vi "NEO VI Example.vi"() -> ()   [LabVIEW 2009]
panel:
  out "msg read?":bool
  out "sn":string
  out "DeviceType:":i32(ring)=65535 items=["NEODEVICE_BLUE"=1, "NEODEVICE_DW_VCAN"=4, "NEODEVICE_FIRE"=8, "NEODEVICE_VCAN3"=16, "NEODEVICE_YELLOW"=32, "NEODEVICE_ALL"=65535]
  out "Number Read:":i32
  out "Number Errors:":i32
  out "Error Info":string
  in  "Get Errors":bool
  out "Msgs":string
  in  "AutoRead":bool
  in  "Wait with Timeout":bool
  in  "Get Messages":bool
  in  "Data":u8[](array[numeric]) format="%.0x"
  in  "Transmit":bool
  in  "Number of \nData Bytes":i32(ring)=8 items=["0", "1", "2", "3", "4", "5", "6", "7", "8", "9", "10", "11"]
  in  "Send Extended ID":bool
  in  "Arb ID":u32 format="%.0x"
  in  "Network":T1(ring)
  in  "Tab Control":enum32{"Quick Set", "Advanced"}(tab)
  in  "Set Bit Rate":bool
  in  "Bit Rate":i32(ring)=20000 items=["20000"=20000, "33333"=33333, "50000"=50000, "62500"=62500, "83333"=83333, "100000"=100000, "125000"=125000, "250000"=250000, "500000"=500000, "800000"=800000, "1000000"=1000000]
  in  "CAN Channel":T2(ring)
  in  "Tab Control 2":enum32{"BLUE, VCAN2, Pro", "FIRE, Red, VCAN3"}(tab)
  in  "Send HS CAN information":bool
  in  "Set HS CAN 250":bool
  in  "Set HS CAN 500":bool
  in  "CNF3":u8 format="%.0x"
  in  "CNF2":u8 format="%.0x"
  in  "CNF1":u8 format="%.0x"
  out "Configuration":string
  in  "Get Configuration":bool
  in  "BRP":u16
  in  "Sync Jump Width":u8
  in  "Propagation Delay":u8
  in  "Phase Segment 2":u8
  in  "Phase Segment 1":u8
  in  "Set 3G Settings":bool
  in  "Get 3G settings":bool
  in  "Get DLL version":bool
  out "status":string
  in  "Close Open Device":bool
  in  "Open First Device":bool
  # "Connection"
  # "Baud Rate"
  # "Transmit Message"
  # "Data in Hex"
  # "Receive Message"
  # "Tip: Use neoVI explorer to get the proper CNFs.\nValueCAN CNFs are different than neoVI due to\ndifferent CAN Chip speeds."
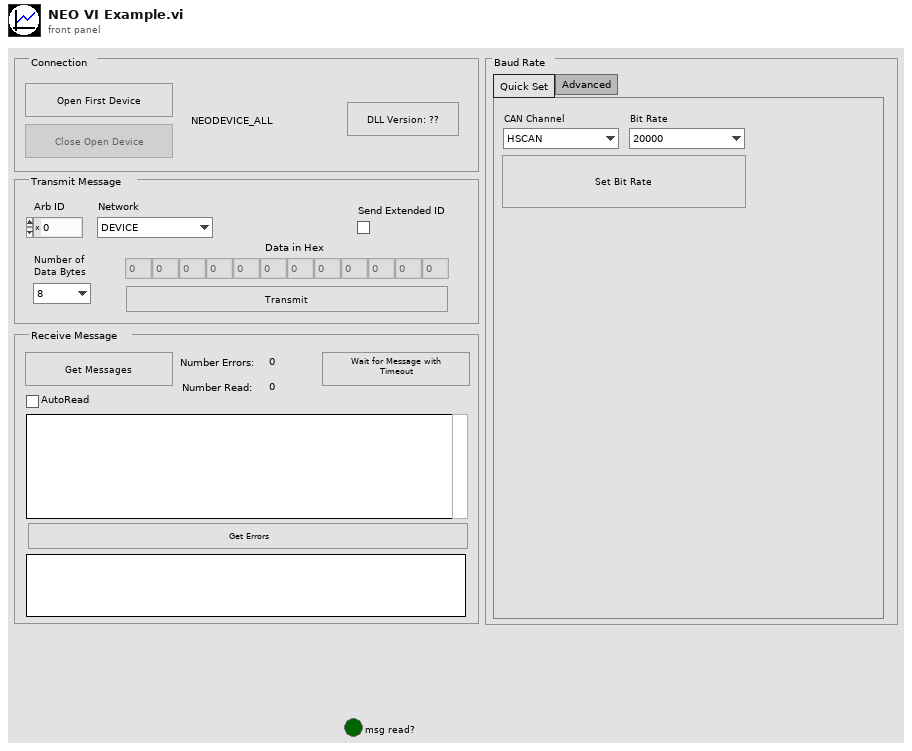
[diagram p1: front panel]
types:
  T1 = enum16{"DEVICE", "HSCAN", "MSCAN", "SWCAN", "LSFTCAN", "FORDSCP", "J1708", "JVPW", "ISO", "FIRE_HSCAN2", "FIRE_MSCAN1", "FIRE_HSCAN3", "FIRE_LIN2", "FIRE_LIN3", "FIRE_LIN4"}
  T2 = enum16{"HSCAN", "MSCAN", "SWCAN", "LSFTCAN", "HSCAN2", "HSCAN3"}
  T3 = enum8{"Enabled", "Disabled", "Disabled and Grayed Out"}
  T4 = cluster{"DeviceType":i32, "Handle":i32, "NumberOfClients":i32, "SerialNumber":i32, "MaxAllowedClients":i32}[]
  T5 = cluster{"DeviceType":i32, "Handle":i32, "NumberOfClients":i32, "SerialNumber":i32, "MaxAllowedClients":i32}
  T6 = typedef "ctl FireSetting.ctl" = cluster{"can 1":cluster{"Mode":u8, "SetBaudrate":u8, "Baudrate":u8, "NetworkType":u8, "TqSeg1":u8, "TqSeg2":u8, "TqProp":u8, "TqSync":u8, "BRP":u16, "auto_baud":u16}, "can 2":cluster{"Mode":u8, "SetBaudrate":u8, "Baudrate":u8, "NetworkType":u8, "TqSeg1":u8, "TqSeg2":u8, "TqProp":u8, "TqSync":u8, "BRP":u16, "auto_baud":u16}, "can 3":cluster{"Mode":u8, "SetBaudrate":u8, "Baudrate":u8, "NetworkType":u8, "TqSeg1":u8, "TqSeg2":u8, "TqProp":u8, "TqSync":u8, "BRP":u16, "auto_baud":u16}, "can 4":cluster{"Mode":u8, "SetBaudrate":u8, "Baudrate":u8, "NetworkType":u8, "TqSeg1":u8, "TqSeg2":u8, "TqProp":u8, "TqSync":u8, "BRP":u16, "auto_baud":u16}, "swcan":cluster{"Mode":u8, "SetBaudrate":u8, "Baudrate":u8, "NetworkType":u8, "TqSeg1":u8, "TqSeg2":u8, "TqProp":u8, "TqSync":u8, "BRP":u16, "high_speed_auto_switch":u16, "auto_baud":u16}, "lsftcan":cluster{"Mode":u8, "SetBaudrate":u8, "Baudrate":u8, "NetworkType":u8, "TqSeg1":u8, "TqSeg2":u8, "TqProp":u8, "TqSync":u8, "BRP":u16, "auto_baud":u16}, "lin 1":cluster{"Baudrate":u32, "spbrg":u16, "brgh":u16, "MasterResistor":u8, "Mode":u8}, "lin 2":cluster{"Baudrate":u32, "spbrg":u16, "brgh":u16, "MasterResistor":u8, "Mode":u8}, "lin 3":cluster{"Baudrate":u32, "spbrg":u16, "brgh":u16, "MasterResistor":u8, "Mode":u8}, "lin 4":cluster{"Baudrate":u32, "spbrg":u16, "brgh":u16, "MasterResistor":u8, "Mode":u8}, "cgi_enable":u16, "cgi_baud":u16, "cgi_tx_ifs_bit_times":u16, "cgi_rx_ifs_bit_times":u16, "cgi_chksum_enable":u16, "network_enalbes":u16, "network_enabled_on_boot":u16, "pwm_man_timeout":u16, "pwm_man_enable":u16, "misc_io_initial_ddr":u16, "misc_io_initial_latch":u16, "misc_io_analog_enable":u16, "misc_io_report_period":u16, "misc_io_on_report_events":u16, "ain_sample_period":u16, "ain_threshold":u16, "iso15765_separation_time_offset":u16, "iso9141_kwp_enable":u16, "ISO9141_Settings":cluster{"Baudrate":u32, "spbrg":u16, "brgh":u16, "ISO9141_KEYWORD2000_INIT_STEP":cluster{"time_500us":u16, "k":u16, "l":u16}, "init_step_count":u8, "p2_500us":u16, "p3_500us":u16, "p4_500us":u16, "chksum_enabled":u16}, "perf_en":u16, "iso_parity":u16, "iso_msg_termination":u16, "iso_tester_pullup_enable":u16, "network_enables_2":u16, "ISO9141__Settings2":cluster{"Baudrate":u32, "spbrg":u16, "brgh":u16, "ISO9141_KEYWORD2000_INIT_STEP":cluster{"time_500us":u16, "k":u16, "l":u16}, "init_step_count":u8, "p2_500us":u16, "p3_500us":u16, "p4_500us":u16, "chksum_enabled":u16}, "iso_parity_2":u16, "iso_msg_termination_2":u16, "ISO9141_Settings_3":cluster{"Baudrate":u32, "spbrg":u16, "brgh":u16, "ISO9141_KEYWORD2000_INIT_STEP":cluster{"time_500us":u16, "k":u16, "l":u16}, "init_step_count":u8, "p2_500us":u16, "p3_500us":u16, "p4_500us":u16, "chksum_enabled":u16}, "iso_parity_3":u16, "iso_msg_termination_3":u16, "ISO9141_Settings_4":cluster{"Baudrate":u32, "spbrg":u16, "brgh":u16, "ISO9141_KEYWORD2000_INIT_STEP":cluster{"time_500us":u16, "k":u16, "l":u16}, "init_step_count":u8, "p2_500us":u16, "p3_500us":u16, "p4_500us":u16, "chksum_enabled":u16}, "iso_parity_4":u16, "iso_msg_termination_4":u16}
  T7 = typedef "ctl SVCANSetting.ctl" = cluster{"can 1":cluster{"Mode":u8, "SetBaudrate":u8, "Baudrate":u8, "NetworkType":u8, "TqSeg1":u8, "TqSeg2":u8, "TqProp":u8, "TqSync":u8, "BRP":u16, "auto_baud":u16}, "can 2":cluster{"Mode":u8, "SetBaudrate":u8, "Baudrate":u8, "NetworkType":u8, "TqSeg1":u8, "TqSeg2":u8, "TqProp":u8, "TqSync":u8, "BRP":u16, "auto_baud":u16}, "network_enables":u16, "network_enabled_on_boot":u16, "iso15765_separation_time_offset":i16, "perf_en":u16, "misc_io_initial_ddr":u16, "misc_io_initial_latach":u16, "misc_io_report_period":u16, "misc_io_on_report_events":u16}
  T8 = typedef "ctl spymessage.ctl" = cluster{"StatusBitField":u32, "StatusBitField2":u32, "TimeHardware":u32, "TimeHardware2":u32, "TimeSystem":u32, "TimeSystem2":u32, "TimeStampHardwareID":u8, "TimeStampHardwareID2":u8, "NetworkID":u8, "NodeID":u8, "Protocol":u8, "MessagePieceID":u8, "ColorID":u8, "NumberBytesHeader":u8, "NumberBytesData":u8, "DescriptionID":u16, "ArbIDOrHeader":u32, "Data [8]":u8[], "AckBytes [8]":u8[], "Value":sgl, "MiscData":u8}
  T9 = enum16{"No Error", "Critical", "Important", "Warning", "Unknown"}
  T10 = cluster{"ErrorNumber":i32, "short":string, "long":string}
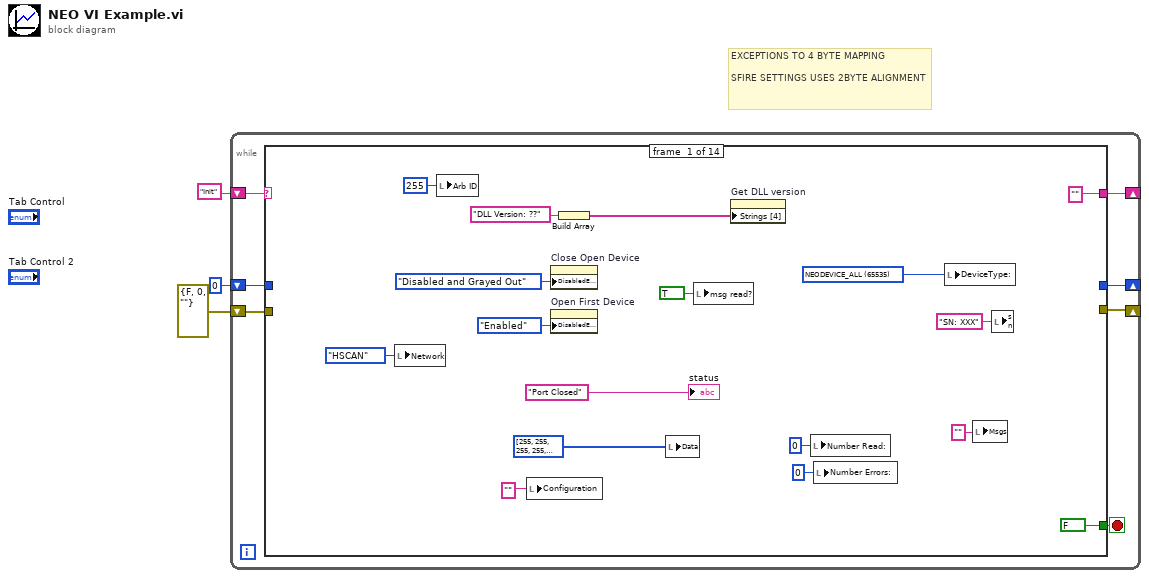
[diagram p0: block diagram]
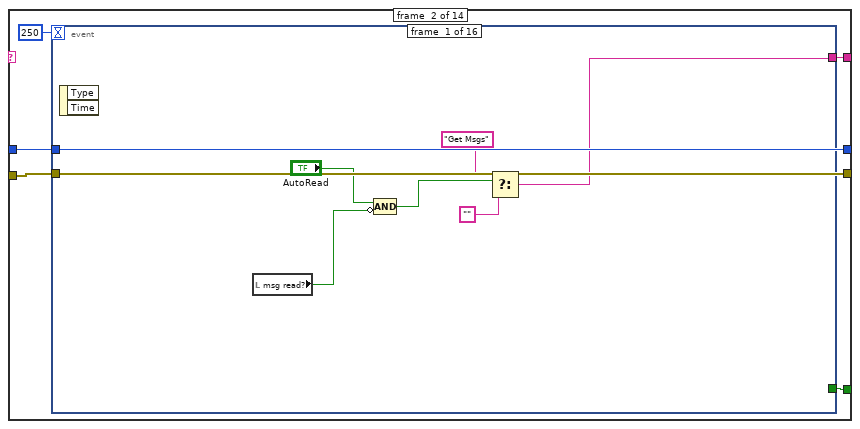
[diagram p2: hidden frame]
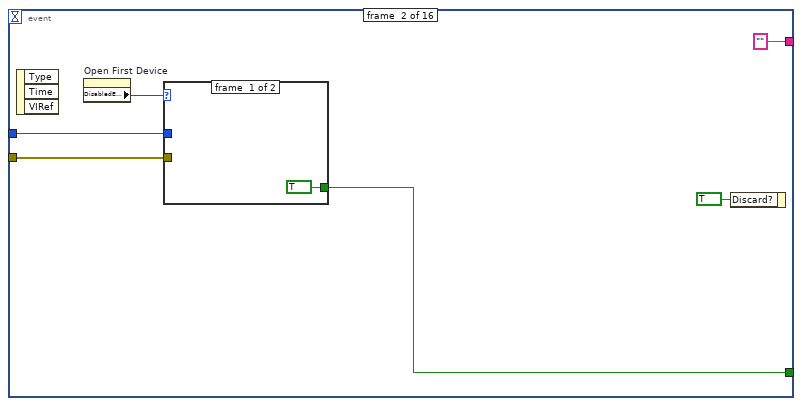
[diagram p3: hidden frame]
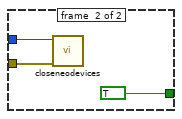
[diagram p4: hidden frame]
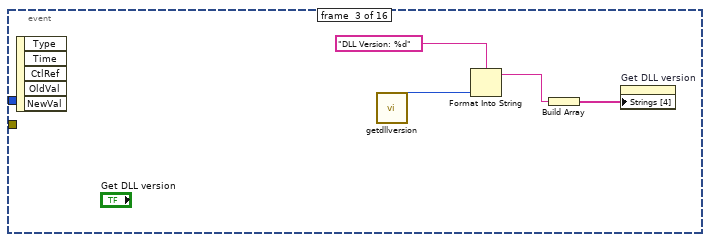
[diagram p5: hidden frame]
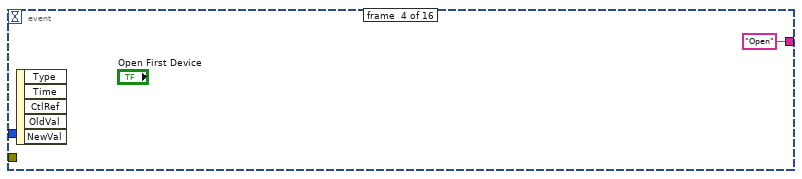
[diagram p6: hidden frame]
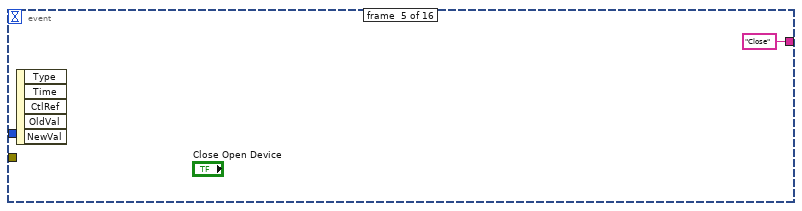
[diagram p7: hidden frame]
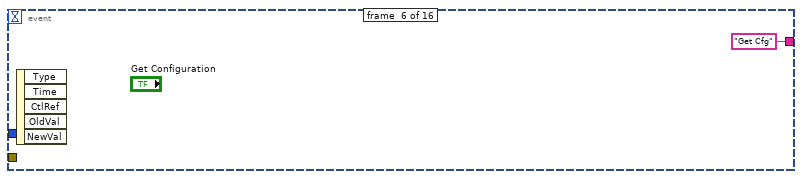
[diagram p8: hidden frame]
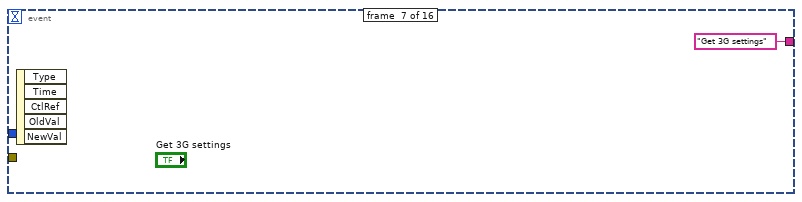
[diagram p9: hidden frame]
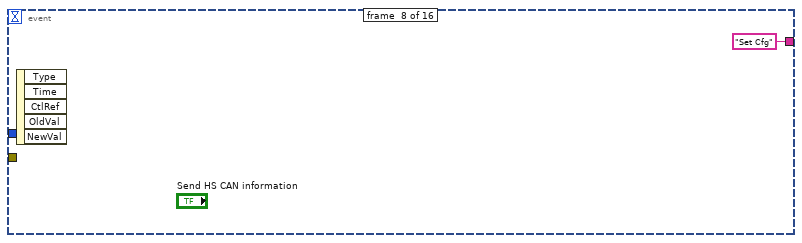
[diagram p10: hidden frame]
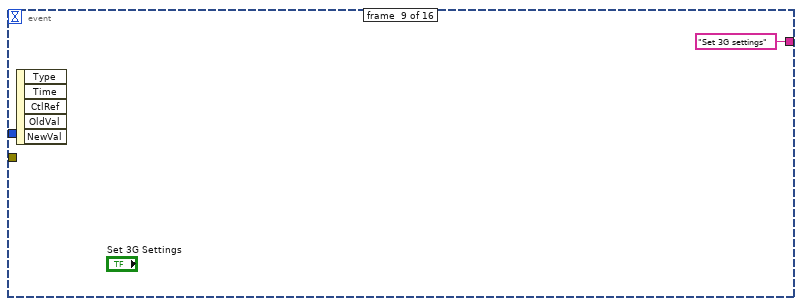
[diagram p11: hidden frame]
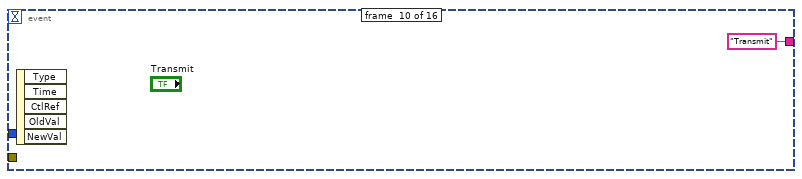
[diagram p12: hidden frame]
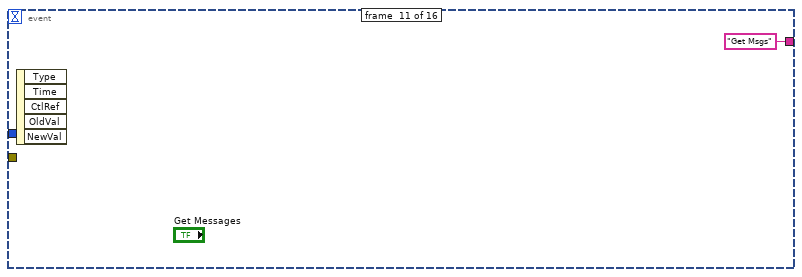
[diagram p13: hidden frame]
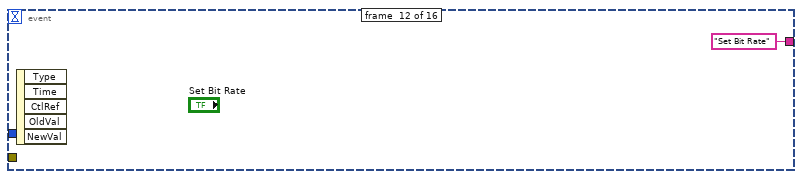
[diagram p14: hidden frame]
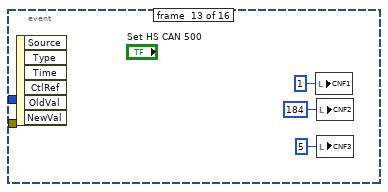
[diagram p15: hidden frame]
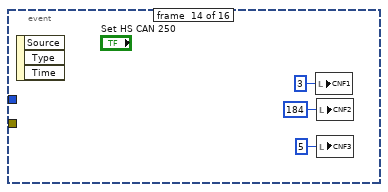
[diagram p16: hidden frame]
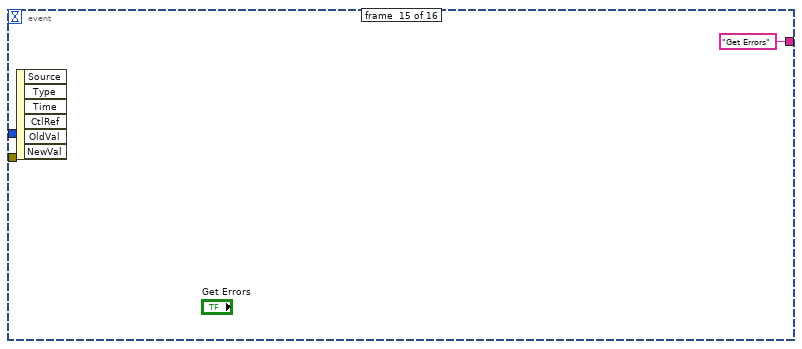
[diagram p17: hidden frame]
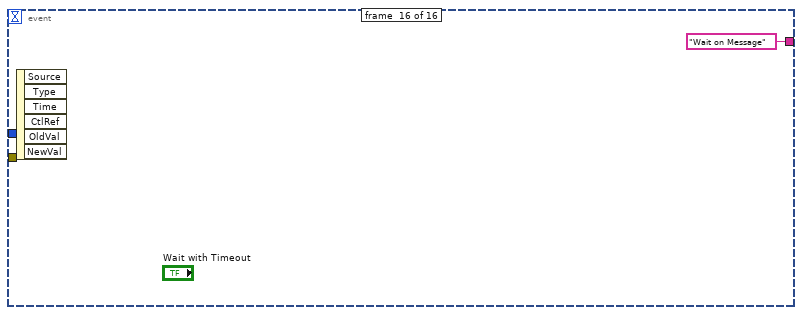
[diagram p18: hidden frame]
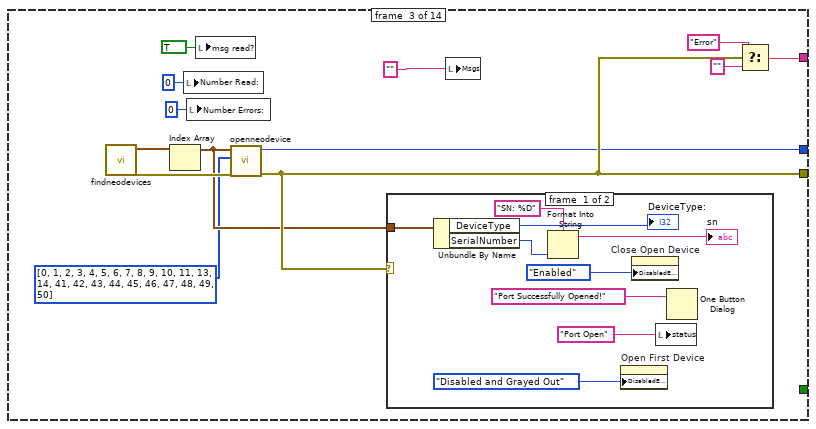
[diagram p19: hidden frame]
diagram:
  # "EXCEPTIONS TO 4 BYTE MAPPING\n\nSFIRE SETTINGS USES 2BYTE ALIGNMENT"
  n1 = while {
    shift-right: [w8] -> _
    shift-left: "Init" -> [w9]
    shift-right: [w7] -> _
    shift-left: 0 ("hObject") -> [w6]
    shift-right: [w5] -> _
    shift-left: errorcluster {"status"=FALSE, "code"=0, "source"=""} ("error out") -> [w4]
    stop <- w10 stop-if-true
    n2 = case shown="\"Open\"" w9 {
      tunnel: [FALSE w32 _ _ _ _ _ _ _ _ _ _ _ _] -> w10
      tunnel: ["" w31 w82 w98 "" ("f") w132 w151 w173 w213 w253 w275 "" ("f") _ _] -> w8
      tunnel: [_ w29 w75 _ w111 w129 w159 w174 w211 w248 w272 0 ("hObject") w291 w318] -> w7
      tunnel: w6 -> [_ w29 _ w94 w110 w142 w158 w179 w204 w258 w279 _ w292 w325]
      tunnel: [_ w28 w79 w95 w112 w128 w152 w175 w212 w254 w270 errorcluster {"status"=FALSE, "code"=0, "source"=""} ("error out") w288 w319] -> w5
      tunnel: w4 -> [_ w28 _ w93 w113 w143 w160 w178 w205 w259 w280 _ w293 w324]
      frame #0 {
        w19 = 65535 items=["NEODEVICE_BLUE"=1, "NEODEVICE_DW_VCAN"=4, "NEODEVICE_FIRE"=8, "NEODEVICE_VCAN3"=16, "NEODEVICE_YELLOW"=32, "NEODEVICE_ALL"=65535] ("DeviceType:")
        n3 = local write "Network"(T1."HSCAN" ("Network")) -> ()
        n4 = local write "Arb ID"(u32 255 ("Arb ID")) -> ()
        n5 = local write "Configuration"("") -> ()
        n6 = property on="Close Open Device" class="Bool"("DisabledEnum"=T3."Disabled and Grayed Out" ("Disabled")) -> ()  [unwired: 2 in, 2 out]
        n7 = property on="Open First Device" class="Bool"("DisabledEnum"=T3."Enabled" ("Disabled")) -> ()  [unwired: 2 in, 2 out]
        n8 = Build Array("DLL Version: ??") -> (w25:string[])
        n9 = local write "Data"(u16[] [255, 255, 255, 255, 255, 255, 255, 255, 255, 255, 255, 255] ("Array")) -> ()
        n10 = local write "msg read?"(TRUE ("msg read?")) -> ()
        n11 = property on="Get DLL version" class="Bool"("Strings [4]"=w25) -> ()  [unwired: 2 in, 2 out]
        n12 = local write "Number Read:"(0 ("Number Read:")) -> ()
        n13 = local write "Number Errors:"(0 ("Number Errors:")) -> ()
        n14 = local write "DeviceType:"(w19) -> ()
        n15 = local write "Msgs"("" ("Msgs")) -> ()
        n16 = local write "sn"("SN: XXX" ("sn")) -> ()
        "status" <- "Port Closed" ("status")
      }
      frame #1 {
        n17 = event shown="[3] \"Open First Device\": Value Change" {
          selector: _ -> [_ _ _ _ _ _ _ _ _ _ _ _ _ _ _ _]
          dyn-events: _ -> [_ _ _ _ _ _ _ _ _ _ _ _ _ _ _ _]
          timeout: 250 -> [_ _ _ _ _ _ _ _ _ _ _ _ _ _ _ _]
          tunnel: [_ w39 _ _ _ _ _ _ _ _ _ _ _ _ _ _] -> w32
          tunnel: [w36 "" _ "Open" "Close" "Get Cfg" "Get 3G settings" "Set Cfg" "Set 3G settings" "Transmit" "Get Msgs" "Set Bit Rate" _ _ "Get Errors" ("f") "Wait on Message" ("f")] -> w31
          tunnel: w29 -> [_ w42 _ _ _ _ _ _ _ _ _ _ _ _ _ _]
          tunnel: w28 -> [_ w41 _ _ _ _ _ _ _ _ _ _ _ _ _ _]
          event #0 {
            n18 = event-data() -> ()  [unwired: 3 out]
            n19 = local read "msg read?"() -> (w33:bool)
            n20 = Compound Arithmetic op=AND("AutoRead", invert w33) -> (w34:bool)
            n21 = Select(t="Get Msgs", s=w34, f="") -> (s? t:f=w36:string)
          }
          event #1 {
            n22 = event-data() -> ()  [unwired: 4 out]
            n23 = property on="Open First Device" class="Bool"() -> ("DisabledEnum"=w40:T3)  [unwired: 2 in, 2 out]
            n24 = case shown="\"Enabled\", Default" w40 {
              tunnel: w42 -> [_ w48]
              tunnel: w41 -> [_ w47]
              tunnel: [TRUE TRUE] -> w39
              frame #0 {
              }
              frame #1 {
                n25 = call "closeneodevices.vi"("error in (no error)"=w47, "hObject"=w48) -> ()  [unwired: 1 in, 9 out]
              }
            }
            n26 = event-data("Discard?"=TRUE) -> ()  [unwired: 1 in, 1 out]
          }
          event #2 {
            n27 = event-data() -> ()  [unwired: 6 out]
            n28 = call "getdllversion.vi"() -> ("DLLVersion"=w52:i32)  [unwired: 1 in, 10 out]
            n29 = Format Into String(format string="DLL Version: %d", w52) -> (resulting string=w50:string)  [unwired: 2 in, 1 out]
            n30 = Build Array(w50) -> (w49:string[])
            n31 = property on="Get DLL version" class="Bool"("Strings [4]"=w49) -> ()  [unwired: 2 in, 2 out]
          }
          event #3 {
            n32 = event-data() -> ()  [unwired: 6 out]
          }
          event #4 {
            n33 = event-data() -> ()  [unwired: 6 out]
          }
          event #5 {
            n34 = event-data() -> ()  [unwired: 6 out]
          }
          event #6 {
            n35 = event-data() -> ()  [unwired: 6 out]
          }
          event #7 {
            n36 = event-data() -> ()  [unwired: 6 out]
          }
          event #8 {
            n37 = event-data() -> ()  [unwired: 6 out]
          }
          event #9 {
            n38 = event-data() -> ()  [unwired: 6 out]
          }
          event #10 {
            n39 = event-data() -> ()  [unwired: 6 out]
          }
          event #11 {
            n40 = event-data() -> ()  [unwired: 6 out]
          }
          event #12 {
            n41 = event-data() -> ()  [unwired: 7 out]
            n42 = local write "CNF1"(u8 1 ("CNF1")) -> ()
            n43 = local write "CNF2"(u8 184 ("CNF2")) -> ()
            n44 = local write "CNF3"(u8 5 ("CNF3")) -> ()
          }
          event #13 {
            n45 = event-data() -> ()  [unwired: 4 out]
            n46 = local write "CNF1"(u8 3 ("CNF1")) -> ()
            n47 = local write "CNF2"(u8 184 ("CNF2")) -> ()
            n48 = local write "CNF3"(u8 5 ("CNF3")) -> ()
          }
          event #14 {
            n49 = event-data() -> ()  [unwired: 7 out]
          }
          event #15 {
            n50 = event-data() -> ()  [unwired: 7 out]
          }
        }
      }
      frame #2 {
        w70 = i8[] [0, 1, 2, 3, 4, 5, 6, 7, 8, 9, 10, 11, 13, 14, 41, 42, 43, 44, 45, 46, 47, 48, 49, 50] items=["NETID_DEVICE"=0, "NETID_HSCAN"=1, "NETID_MSCAN"=2, "NETID_SWCAN"=3, "NETID_LSFTCAN"=4, "NETID_FORDSCP"=5, "NETID_J1708"=6, "NETID_AUX"=7, "NETID_JVPW"=8, "NETID_ISO_LIN"=9, "NETID_ISOPIC"=10, "NETID_MAIN51"=11, "NETID_SCI"=13, "NETID_ISO2"=14, "NETID_FIRE_HSCAN1"=41, "NETID_FIRE_HSCAN2"=42, "NETID_FIRE_MSCAN1"=43, "NETID_FIRE_MSCAN2_HSCAN3"=44, "NETID_FIRE_SWCAN"=45, "NETID_FIRE_LSFT"=46, "NETID_FIRE_LIN1"=47, "NETID_FIRE_LIN2"=48, "NETID_FIRE_LIN3"=49, "NETID_FIRE_LIN4"=50] ("bNetworkIDs")
        n51 = call "findneodevices.vi"() -> ("error out"=w77:errorcluster, "NeoDevices {}"=w78:T4)  [unwired: 3 in, 7 out]
        n52 = Index Array(array=w78) -> (element=w76:T5)  [unwired: 1 in]
        n53 = local write "Number Read:"(0 ("Number Read:")) -> ()
        n54 = local write "Number Errors:"(0 ("Number Errors:")) -> ()
        n55 = local write "msg read?"(TRUE ("msg read?")) -> ()
        n56 = call "openneodevice.vi"("error in (no error)"=w77, "bNetworkIDs"=w70, "NeoDevice{}"=w76) -> ("error out"=w79:errorcluster, "hObject"=w75:i32)  [unwired: 2 in, 5 out]
        n57 = case shown="No Error" w79 {
          tunnel: w76 -> [w87 _]
          frame #0 {
            n58 = Unbundle By Name(w87) -> ("DeviceType"=→"DeviceType:":i32, "SerialNumber"=w85:i32)
            n59 = Format Into String(format string="SN: %D", w85) -> (resulting string=→"sn":string)  [unwired: 2 in, 1 out]
            n60 = property on="Open First Device" class="Bool"("DisabledEnum"=T3."Disabled and Grayed Out" ("Disabled")) -> ()  [unwired: 2 in, 2 out]
            n61 = property on="Close Open Device" class="Bool"("DisabledEnum"=T3."Enabled" ("Disabled")) -> ()  [unwired: 2 in, 2 out]
            n62 = local write "status"("Port Open" ("status")) -> ()
            n63 = One Button Dialog(message="Port Successfully Opened!") -> ()  [unwired: 2 out]
          }
          frame #1 {
          }
        }
        n64 = local write "Msgs"("" ("Msgs")) -> ()
        n65 = Select(t="Error", s=w79, f="") -> (s? t:f=w82:string)
      }
      frame #3 {
        n66 = local write "msg read?"(TRUE ("msg read?")) -> ()
        n67 = call "closeneodevices.vi"("error in (no error)"=w93, "hObject"=w94) -> ("error out"=w95:errorcluster)  [unwired: 1 in, 8 out]
        n68 = case shown="No Error" w95 {
          frame #0 {
            w100 = 65535 items=["NEODEVICE_BLUE"=1, "NEODEVICE_DW_VCAN"=4, "NEODEVICE_FIRE"=8, "NEODEVICE_VCAN3"=16, "NEODEVICE_YELLOW"=32, "NEODEVICE_ALL"=65535] ("DeviceType:")
            n69 = local write "sn"("SN: XXX" ("sn")) -> ()
            n70 = property on="Open First Device" class="Bool"("DisabledEnum"=T3."Enabled" ("Disabled")) -> ()  [unwired: 2 in, 2 out]
            n71 = local write "status"("Port Closed" ("status")) -> ()
            n72 = local write "DeviceType:"(w100) -> ()
            n73 = property on="Close Open Device" class="Bool"("DisabledEnum"=T3."Disabled and Grayed Out" ("Disabled")) -> ()  [unwired: 2 in, 2 out]
          }
          frame #1 {
          }
        }
        n74 = Select(t="Error", s=w95, f="") -> (s? t:f=w98:string)
      }
      frame #4 {
        n75 = call "getconfiguration.vi"("error in (no error)"=w113, "hObject"=w110) -> ("error out"=w112:errorcluster, "pINumBytes"=w105:i32, "pData"=w109:u8[], "hObject Out"=w111:i32)  [unwired: 6 out]
        n76 = for {
          N: w105 -> [_]
          tunnel: w109 -> [w118] mode=indexing
          tunnel: "Byte %d: %d " ("format string") -> [w120]
          shift-right: [w114] -> w106
          shift-left: "" -> [w117]
          i -> [w119]
          n77 = Format Into String(format string=w120, w119, w118) -> (resulting string=w116:string)  [unwired: 2 in, 1 out]
          n78 = Concatenate Strings(w117, w116, "\r") -> (w114:string)
        }
        "Configuration" <- w106
      }
      frame #5 {
        n79 = call "getconfiguration.vi"("error in (no error)"=w143, "hObject"=w142) -> ("error out"=w141:errorcluster, "pData"=w136:u8[], "hObject Out"=w140:i32)  [unwired: 7 out]
        n80 = Replace Array Subset(array=w136, new element #1="CNF1", index #1=522 ("index"), new element #2="CNF2", index #2=521 ("index"), new element #3="CNF3", index #3=520 ("index")) -> (w135:u8[])
        n81 = call "sendconfiguration.vi"("error in (no error)"=w141, "pData"=w135, "hObject"=w140) -> ("error out"=w131:errorcluster, "hObject Out"=w130:i32)  [unwired: 7 out]
        n82 = call "getconfiguration.vi"("error in (no error)"=w131, "hObject"=w130) -> ("error out"=w128:errorcluster, "pData"=w125:u8[], "hObject Out"=w129:i32)  [unwired: 7 out]
        n83 = for {
          tunnel: w125 -> [w148] mode=indexing
          tunnel: "Byte %d: %d " ("format string") -> [w150]
          shift-right: [w144] -> w124
          shift-left: "" -> [w147]
          i -> [w149]
          n84 = Format Into String(format string=w150, w149, w148) -> (resulting string=w146:string)  [unwired: 2 in, 1 out]
          n85 = Concatenate Strings(w147, w146, "\r") -> (w144:string)
        }
        n86 = local write "Configuration"(w124) -> ()
        n87 = Select(t="Error", s=w128, f="") -> (s? t:f=w132:string)
      }
      frame #6 {
        n88 = case shown="\"HSCAN3\"" "CAN Channel" {
          tunnel: [_ w161 w162 w163 w164 w165 w166] -> w155
          frame #0 {
          }
          frame #1 {
            w161 = i8 1 items=["NETID_DEVICE"=0, "NETID_HSCAN"=1, "NETID_MSCAN"=2, "NETID_SWCAN"=3, "NETID_LSFTCAN"=4, "NETID_FORDSCP"=5, "NETID_J1708"=6, "NETID_AUX"=7, "NETID_JVPW"=8, "NETID_ISO_LIN"=9, "NETID_ISOPIC"=10, "NETID_MAIN51"=11, "NETID_SCI"=13, "NETID_ISO2"=14, "NETID_FIRE_HSCAN1"=41, "NETID_FIRE_HSCAN2"=42, "NETID_FIRE_MSCAN1"=43, "NETID_FIRE_MSCAN2_HSCAN3"=44, "NETID_FIRE_SWCAN"=45, "NETID_FIRE_LSFT"=46, "NETID_FIRE_LIN1"=47, "NETID_FIRE_LIN2"=48, "NETID_FIRE_LIN3"=49, "NETID_FIRE_LIN4"=50] ("NetworkID")
          }
          frame #2 {
            w162 = i8 2 items=["NETID_DEVICE"=0, "NETID_HSCAN"=1, "NETID_MSCAN"=2, "NETID_SWCAN"=3, "NETID_LSFTCAN"=4, "NETID_FORDSCP"=5, "NETID_J1708"=6, "NETID_AUX"=7, "NETID_JVPW"=8, "NETID_ISO_LIN"=9, "NETID_ISOPIC"=10, "NETID_MAIN51"=11, "NETID_SCI"=13, "NETID_ISO2"=14, "NETID_FIRE_HSCAN1"=41, "NETID_FIRE_HSCAN2"=42, "NETID_FIRE_MSCAN1"=43, "NETID_FIRE_MSCAN2_HSCAN3"=44, "NETID_FIRE_SWCAN"=45, "NETID_FIRE_LSFT"=46, "NETID_FIRE_LIN1"=47, "NETID_FIRE_LIN2"=48, "NETID_FIRE_LIN3"=49, "NETID_FIRE_LIN4"=50] ("NetworkID")
          }
          frame #3 {
            w163 = i8 3 items=["NETID_DEVICE"=0, "NETID_HSCAN"=1, "NETID_MSCAN"=2, "NETID_SWCAN"=3, "NETID_LSFTCAN"=4, "NETID_FORDSCP"=5, "NETID_J1708"=6, "NETID_AUX"=7, "NETID_JVPW"=8, "NETID_ISO_LIN"=9, "NETID_ISOPIC"=10, "NETID_MAIN51"=11, "NETID_SCI"=13, "NETID_ISO2"=14, "NETID_FIRE_HSCAN1"=41, "NETID_FIRE_HSCAN2"=42, "NETID_FIRE_MSCAN1"=43, "NETID_FIRE_MSCAN2_HSCAN3"=44, "NETID_FIRE_SWCAN"=45, "NETID_FIRE_LSFT"=46, "NETID_FIRE_LIN1"=47, "NETID_FIRE_LIN2"=48, "NETID_FIRE_LIN3"=49, "NETID_FIRE_LIN4"=50] ("NetworkID")
          }
          frame #4 {
            w164 = i8 4 items=["NETID_DEVICE"=0, "NETID_HSCAN"=1, "NETID_MSCAN"=2, "NETID_SWCAN"=3, "NETID_LSFTCAN"=4, "NETID_FORDSCP"=5, "NETID_J1708"=6, "NETID_AUX"=7, "NETID_JVPW"=8, "NETID_ISO_LIN"=9, "NETID_ISOPIC"=10, "NETID_MAIN51"=11, "NETID_SCI"=13, "NETID_ISO2"=14, "NETID_FIRE_HSCAN1"=41, "NETID_FIRE_HSCAN2"=42, "NETID_FIRE_MSCAN1"=43, "NETID_FIRE_MSCAN2_HSCAN3"=44, "NETID_FIRE_SWCAN"=45, "NETID_FIRE_LSFT"=46, "NETID_FIRE_LIN1"=47, "NETID_FIRE_LIN2"=48, "NETID_FIRE_LIN3"=49, "NETID_FIRE_LIN4"=50] ("NetworkID")
          }
          frame #5 {
            w165 = i8 42 items=["NETID_DEVICE"=0, "NETID_HSCAN"=1, "NETID_MSCAN"=2, "NETID_SWCAN"=3, "NETID_LSFTCAN"=4, "NETID_FORDSCP"=5, "NETID_J1708"=6, "NETID_AUX"=7, "NETID_JVPW"=8, "NETID_ISO_LIN"=9, "NETID_ISOPIC"=10, "NETID_MAIN51"=11, "NETID_SCI"=13, "NETID_ISO2"=14, "NETID_FIRE_HSCAN1"=41, "NETID_FIRE_HSCAN2"=42, "NETID_FIRE_MSCAN1"=43, "NETID_FIRE_MSCAN2_HSCAN3"=44, "NETID_FIRE_SWCAN"=45, "NETID_FIRE_LSFT"=46, "NETID_FIRE_LIN1"=47, "NETID_FIRE_LIN2"=48, "NETID_FIRE_LIN3"=49, "NETID_FIRE_LIN4"=50] ("NetworkID")
          }
          frame #6 {
            w166 = i8 44 items=["NETID_DEVICE"=0, "NETID_HSCAN"=1, "NETID_MSCAN"=2, "NETID_SWCAN"=3, "NETID_LSFTCAN"=4, "NETID_FORDSCP"=5, "NETID_J1708"=6, "NETID_AUX"=7, "NETID_JVPW"=8, "NETID_ISO_LIN"=9, "NETID_ISOPIC"=10, "NETID_MAIN51"=11, "NETID_SCI"=13, "NETID_ISO2"=14, "NETID_FIRE_HSCAN1"=41, "NETID_FIRE_HSCAN2"=42, "NETID_FIRE_MSCAN1"=43, "NETID_FIRE_MSCAN2_HSCAN3"=44, "NETID_FIRE_SWCAN"=45, "NETID_FIRE_LSFT"=46, "NETID_FIRE_LIN1"=47, "NETID_FIRE_LIN2"=48, "NETID_FIRE_LIN3"=49, "NETID_FIRE_LIN4"=50] ("NetworkID")
          }
        }
        n89 = call "setbitrate.vi"("error in (no error)"=w160, "NetworkID"=w155, "BitRate"="Bit Rate", "hObject"=w158) -> ("error out"=w152:errorcluster, "hObject Out"=w159:i32)  [unwired: 6 out]
        n90 = Select(t="Error", s=w152, f="") -> (s? t:f=w151:string)
      }
      frame #7 {
        n91 = local read "DeviceType:"() -> (w167:i32)
        n92 = case shown="16" w167 {
          tunnel: w179 -> [w181 w192 w202]
          tunnel: w178 -> [w182 w191 w201]
          tunnel: [w182 w190 w200] -> w175
          tunnel: [w181 w189 w199] -> w174
          tunnel: [_ w187 w197] -> w172
          tunnel: [_ w186 w196] -> w171
          tunnel: [_ w185 w195] -> w170
          tunnel: [_ w184 w194] -> w169
          tunnel: [_ w183 w193] -> w168
          frame #0 {
            n93 = One Button Dialog(message="Problem reading configuration, unsupported device") -> ()  [unwired: 2 out]
          }
          frame #1 {
            n94 = call "getfiresettings.vi"("error in (no error)"=w191, "hObject"=w192) -> ("error out"=w190:errorcluster, "pSettings"=w188:T6, "hObject Out"=w189:i32)  [unwired: 7 out]
            n95 = Unbundle By Name(w188) -> ("can 1.TqSeg1"=w187:u8, "can 1.TqSeg2"=w186:u8, "can 1.TqProp"=w185:u8, "can 1.TqSync"=w184:u8, "can 1.BRP"=w183:u16)
          }
          frame #2 {
            n96 = call "getvcan3setting.vi"("error in (no error)"=w201, "hObject"=w202) -> ("error out"=w200:errorcluster, "SVCAN3Setting"=w198:T7, "hObject Out"=w199:i32)  [unwired: 7 out]
            n97 = Unbundle By Name(w198) -> ("can 1.TqSeg1"=w197:u8, "can 1.TqSeg2"=w196:u8, "can 1.TqProp"=w195:u8, "can 1.TqSync"=w194:u8, "can 1.BRP"=w193:u16)
          }
        }
        n98 = local write "Phase Segment 1"(w172) -> ()
        n99 = local write "Phase Segment 2"(w171) -> ()
        n100 = local write "Propagation Delay"(w170) -> ()
        n101 = local write "Sync Jump Width"(w169) -> ()
        n102 = local write "BRP"(w168) -> ()
        n103 = Select(t="Error", s=w175, f="") -> (s? t:f=w173:string)
      }
      frame #8 {
        n104 = local read "DeviceType:"() -> (w203:i32)
        n105 = case shown="8" w203 {
          tunnel: [w217 w232 w246] -> w212
          tunnel: [w218 w231 w245] -> w211
          tunnel: "Phase Segment 1" -> [_ w229 w244]
          tunnel: "Phase Segment 2" -> [_ w228 w243]
          tunnel: "Propagation Delay" -> [_ w227 w242]
          tunnel: "Sync Jump Width" -> [_ w226 w241]
          tunnel: "BRP" -> [_ w225 w240]
          tunnel: w205 -> [w217 w224 w239]
          tunnel: w204 -> [w218 w223 w238]
          frame #0 {
            n106 = One Button Dialog(message="Problem sending configuration, unsupported device") -> ()  [unwired: 2 out]
          }
          frame #1 {
            n107 = call "getfiresettings.vi"("error in (no error)"=w224, "hObject"=w223) -> ("error out"=w221:errorcluster, "pSettings"=w220:T6, "hObject Out"=w222:i32)  [unwired: 7 out]
            n108 = Bundle By Name(cluster=w220, "can 1.TqSeg1"=w229, "can 1.TqSeg2"=w228, "can 1.TqProp"=w227, "can 1.TqSync"=w226, "can 1.BRP"=w225, "can 1.SetBaudrate"=u8 1) -> (w230:T6)
            n109 = call "setfiresettings.vi"("error in (no error)"=w221, "firesetting {}"=w230, "hObject"=w222) -> ("error out"=w232:errorcluster, "hObject Out"=w231:i32)  [unwired: 1 in, 6 out]
          }
          frame #2 {
            n110 = call "getvcan3setting.vi"("error in (no error)"=w239, "hObject"=w238) -> ("error out"=w236:errorcluster, "SVCAN3Setting"=w235:T7, "hObject Out"=w237:i32)  [unwired: 7 out]
            n111 = Bundle By Name(cluster=w235, "can 1.TqSeg1"=w244, "can 1.TqSeg2"=w243, "can 1.TqProp"=w242, "can 1.TqSync"=w241, "can 1.BRP"=w240, "can 1.SetBaudrate"=u8 1) -> (w234:T7)
            n112 = call "setvcan3setting.vi"("error in (no error)"=w236, "SVCAN3Setting"=w234, "hObject"=w237) -> ("error out"=w246:errorcluster, "hObject Out"=w245:i32)  [unwired: 7 out]
          }
        }
        n113 = Select(t="Error", s=w212, f="") -> (s? t:f=w213:string)
      }
      frame #9 {
        n114 = call "getmessages.vi"("error in (no error)"=w259, "hObject"=w258) -> ("error out"=w254:errorcluster, "NumMessages"=→"Number Read:":i32, "pMsgs"=w257:T8[], "hObject Out"=w248:i32, "NumOfErrors"=w251:i32)  [unwired: 5 out]
        n115 = for {
          tunnel: w257 -> [w264] mode=indexing
          shift-right: [w260] -> w249
          shift-left: "" -> [w262]
          tunnel: w248 -> [w265]
          n116 = call "GetTimeStampForMsg.vi"("SpyMessage{}"=w264, "hObject"=w265) -> ("pTimeStamp"=w263:dbl)  [unwired: 1 in, 8 out]
          n117 = call "build status string.vi"("SpyMessage{}"=w264, "timestamp"=w263) -> ("string out"=w261:string)  [unwired: 1 in]
          n118 = Concatenate Strings(w262, w261) -> (w260:string)
        }
        "Msgs" <- w249
        n119 = local write "Number Errors:"(w251) -> ()
        n120 = Select(t="Error", s=w254, f="") -> (s? t:f=w253:string)
        "msg read?" <- TRUE ("msg read?")
      }
      frame #10 {
        n121 = call "transmit messages.vi"("extended ID?"="Send Extended ID", "Network"="Network", "Arb ID"="Arb ID", "error in"=w280, "Number of \nData Bytes"="Number of \nData Bytes", "hObject In"=w279, "Data"="Data") -> ("error out"=w271:errorcluster, "hObject Out"=w273:i32)  [unwired: 3 out]
        n122 = local write "msg read?"(FALSE ("msg read?")) -> ()
        n123 = call "geterrormessages.vi"("error in (no error)"=w271, "hObject"=w273) -> ("error out"=w270:errorcluster, "pNumOfErrors"=→"Number Errors:":i32, "hObject Out"=w272:i32)  [unwired: 7 out]
        n124 = Select(t="Error", s=w270, f="") -> (s? t:f=w275:string)
      }
      frame #11 {
        n125 = One Button Dialog(message="Problem occurred communicating with the device") -> ()  [unwired: 2 out]
      }
      frame #12 {
        n126 = call "geterrormessages.vi"("error in (no error)"=w293, "hObject"=w292) -> ("error out"=w290:errorcluster, "pNumOfErrors"=w286:i32, "pErrorMsgs"=w289:i32[], "hObject Out"=w291:i32)  [unwired: 6 in]
        n127 = local write "Number Errors:"(w286) -> ()
        n128 = case shown="0, Default" w286 {
          tunnel: w290 -> [w294 w302]
          tunnel: w289 -> [_ w301]
          tunnel: [w294 w300] -> w288
          tunnel: ["No Errors" w297] -> w287
          frame #0 {
          }
          frame #1 {
            n129 = for {
              shift-right: [w314] -> w300
              shift-left: w302 -> [w315]
              tunnel: w301 -> [w313] mode=indexing
              shift-right: [w304] -> w297
              shift-left: "" -> [w307]
              tunnel: "Error#%d, Short Desc: %s, Long Desc: %s, Severity: %s" ("format string") -> [w308]
              tunnel: "\r" -> [w305]
              n130 = call "GetErrorInfo.vi"("error in (no error)"=w315, "ErrorNumber"=w313) -> ("error out"=w314:errorcluster, "severity"=w303:T9, "Error{}"=w312:T10)  [unwired: 6 in, 1 out]
              n131 = Unbundle By Name(w312) -> ("ErrorNumber"=w311:i32, "short"=w310:string, "long"=w309:string)
              n132 = Format Into String(format string=w308, w311, w310, w309, w303) -> (resulting string=w306:string)  [unwired: 2 in, 1 out]
              n133 = Concatenate Strings(w307, w306, w305) -> (w304:string)
            }
          }
        }
        "Error Info" <- w287
      }
      frame #13 {
        # "Check for messages for 5 seconds"
        n134 = for {
          N: 10 -> [_]
          shift-right: [w347] -> w322
          shift-left: w325 -> [w354]
          shift-right: [w348] -> w320
          shift-left: w324 -> [w353]
          tunnel: [w346] -> w317
          tunnel: [w345] -> w321
          stop <- w349 stop-if-true
          n135 = call "getmessages.vi"("error in (no error)"=w353, "hObject"=w354) -> ("error out"=w348:errorcluster, "NumMessages"=w346:i32, "pMsgs"=w345:T8[], "hObject Out"=w347:i32, "NumOfErrors"=w352:i32)  [unwired: 5 out]
          n136 = Greater Than 0?(x=w346) -> (x > 0?=w351:bool)
          n137 = Greater Than 0?(x=w352) -> (x > 0?=w350:bool)
          n138 = stacked-sequence {
            tunnel: w347 -> [_]
            frame #0 {
              n139 = Wait (ms)(milliseconds to wait=u32 500) -> ()  [unwired: 1 out]
            }
          }
          n140 = Or(x=w351, y=w350) -> (x .or. y?=w349:bool)
        }
        n141 = case shown="1.." w317 {
          tunnel: w322 -> [w327 w334]
          tunnel: w321 -> [_ w333]
          tunnel: w320 -> [w326 w332]
          tunnel: [w326 w331] -> w319
          tunnel: [w327 w330] -> w318
          tunnel: [_ FALSE ("Wait with Timeout")] -> w316
          frame #0 {
          }
          frame #1 {
            n142 = for {
              tunnel: w333 -> [w343] mode=indexing
              shift-right: [w339] -> w329
              shift-left: "" -> [w341]
              tunnel: w334 -> [w344]
              shift-right: [w337] -> w331
              shift-left: w332 -> [w338]
              tunnel: [w336] -> w330
              n143 = call "GetTimeStampForMsg.vi"("error in (no error)"=w338, "SpyMessage{}"=w343, "hObject"=w344) -> ("error out"=w337:errorcluster, "pTimeStamp"=w342:dbl, "hObject Out"=w336:i32)  [unwired: 6 out]
              n144 = call "build status string.vi"("SpyMessage{}"=w343, "timestamp"=w342) -> ("string out"=w340:string)  [unwired: 1 in]
              n145 = Concatenate Strings(w341, w340) -> (w339:string)
            }
            n146 = local write "Msgs"(w329) -> ()
          }
        }
        n147 = local write "Wait with Timeout"(w316) -> ()
      }
    }
  }
